vi "Parse Dependency Information.vi"(8 "error in (no error)":errorcluster, 11 "CustomDeviceVI":refnum<k24>[](array[refnum])) -> (0 "error out":errorcluster, 2 "Dependency Information":T1[](array[typedef]) {"Type" items=["Absolute", "ToBase", "ToCommonDocDir", "ToApplicationDataDir"]}, 3 "CustomDeviceVI":refnum<k24>[](array[refnum]))   [LabVIEW 2020, in "VeriStand SLSC Scripting.lvlib"]
uses:
  VeriStand SLSC Scripting.lvlib
  NationalInstruments.VeriStand.XMLReader
  Controls/Dependent File Information.ctl
  <vilib>/NI VeriStand/Custom Device API/Custom Device Supported Target.ctl
  <vilib>/NI VeriStand/Custom Device API/Custom Device API.lvlib
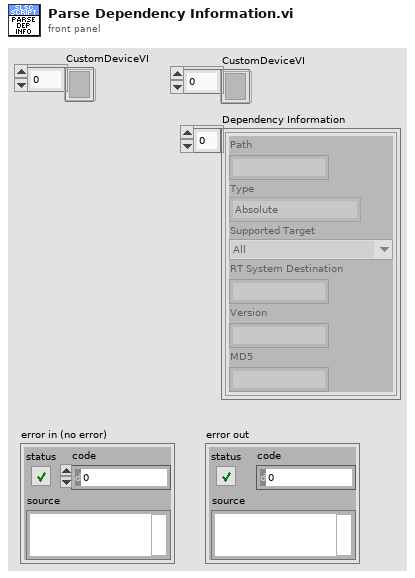
[diagram p1: front panel]
types:
  T1 = typedef "VeriStand SLSC Scripting.lvlib/Dependent File Information.ctl" = cluster{"Path":string, "Type":i32, "Supported Target":T2, "RT System Destination":string, "Version":string, "MD5":string}
  T2 = typedef "Custom Device API.lvlib/Custom Device Supported Target.ctl" = enum16{"All", "PharLap", "VxWorks", "Windows", "Linux_32_ARM", "Linux_x64", "PharLap & Windows", "PharLap & VxWorks", "VxWorks & Windows"}
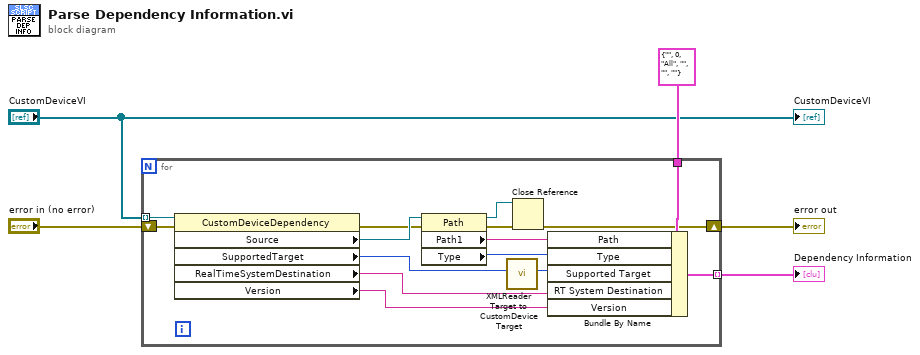
[diagram p0: block diagram]
diagram:
  n1 = for {
    tunnel: "CustomDeviceVI" -> [w20] mode=indexing
    tunnel: T1 {"Path"="", "Type"=0, "Supported Target"=enum."All", "RT System Destination"="", "Version"="", "MD5"=""} ("Driver VI Information") -> [w18]
    tunnel: [w14] -> w4 mode=indexing
    shift-right: [w10] -> w5
    shift-left: "error in (no error)" -> [w13]
    n2 = property class="CustomDeviceDependency"(reference=w20, error in=w13) -> (error out=w12:errorcluster, "Source"=w19:refnum<k24>, "SupportedTarget"=w8:i32, "RealTimeSystemDestination"=w15:string, "Version"=w6:string)  [unwired: 1 out]
    n3 = property class="Path"(reference=w19, error in=w12) -> (reference out=w9:refnum<k24>, error out=w11:errorcluster, "Path1"=w17:string, "Type"=w16:i32)
    n4 = call "XMLReader Target to CustomDevice Target.vi"("XMLReader SupportedTarget"=w8) -> ("CustomDevice Supported Target"=w7:T2)  [unwired: 10 in]
    n5 = Close Reference(reference=w9, error in (no error)=w11) -> (error out=w10:errorcluster)
    n6 = Bundle By Name(cluster=w18, "Path"=w17, "Type"=w16, "Supported Target"=w7, "RT System Destination"=w15, "Version"=w6) -> (w14:T1)
  }
  "error out" <- w5
  "Dependency Information" <- w4
  "CustomDeviceVI" <- "CustomDeviceVI"
